vi "SaveStatMeas.vi"(2 "Min":dbl, 3 "Max":dbl, 4 "error in":errorcluster, 5 "Ecart Type":dbl, 6 "Moyenne":dbl, 7 "storage refnum (file)":refnum<k20>) -> (0 "error out":errorcluster, 1 "storage refnum (file) 2":refnum<k20>)   [LabVIEW 2014]
uses:
  <vilib>/Platform/storage/Storage.llb/usiSequenceRepresentation.ctl
  <vilib>/Platform/storage/Storage.llb/usiOverwriteOptions.ctl
  <vilib>/Platform/storage/lvStorage.llb/_createOrGetByNameExplicitChildObject.vi
  <vilib>/Platform/storage/Storage.llb/__savePropString.vi
  <vilib>/Platform/storage/lvStorage.llb/xStorage/xStorageSupp/ErrorOut.vi
  <vilib>/Platform/storage/lvStorage.llb/__saveFloat64Channel.vi
  <vilib>/Platform/storage/lvStorage.llb/xStorage/Write Data/Write Data.xnode
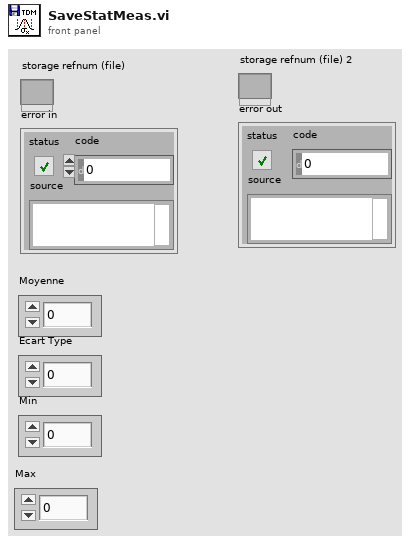
[diagram p1: front panel]
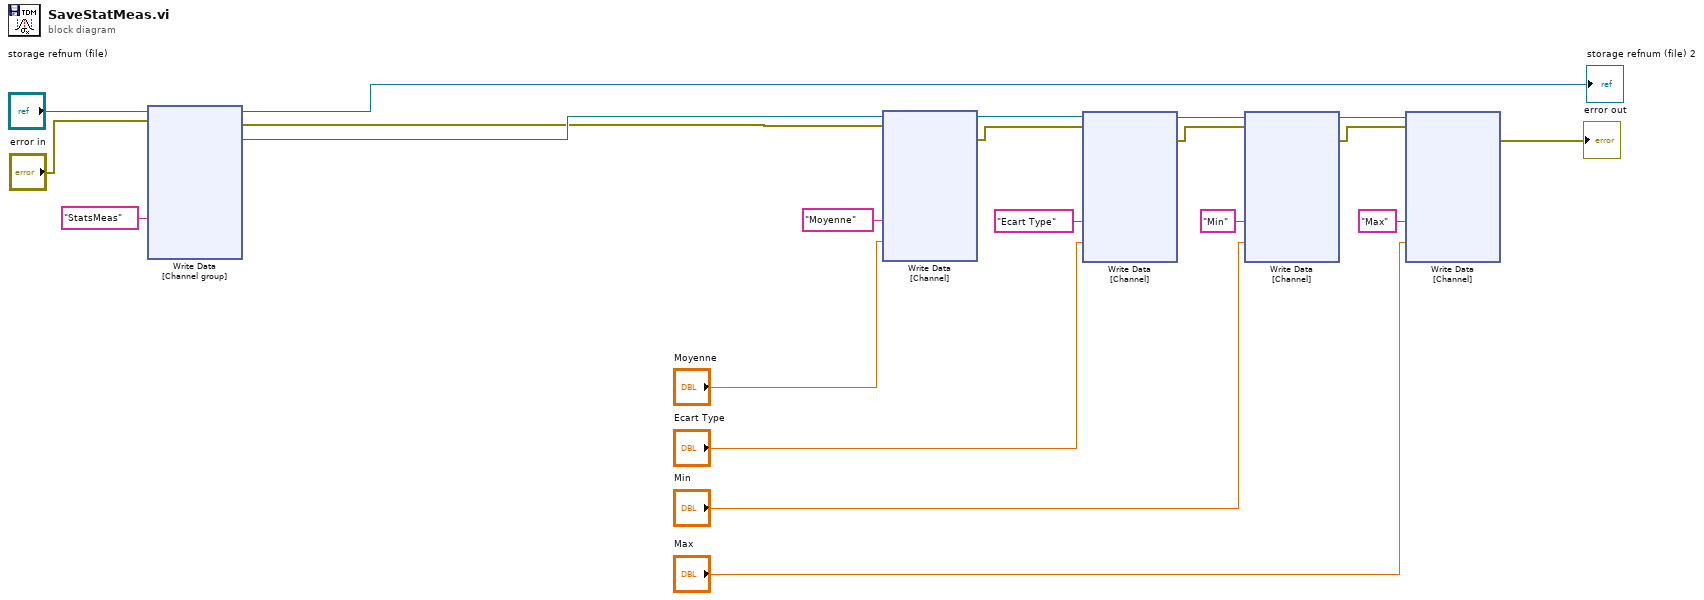
[diagram p0: block diagram]
diagram:
  n1 = xnode "Write Data\n[Channel group]"("Name"="StatsMeas", "storage refnum (file)"="storage refnum (file)", "error in"="error in") -> ("error out"=w17:errorcluster, "storage refnum (channel group)"=w18:refnum<k20>)  [unwired: 1 in, 1 out]
  n2 = xnode "Write Data\n[Channel]"("Name"="Moyenne", "Signal"="Moyenne", "storage refnum (channel group)"=w18, "error in"=w17) -> ("storage refnum (channel group) out"=w11:refnum<k20>, "error out"=w14:errorcluster)  [unwired: 2 in, 1 out]
  n3 = xnode "Write Data\n[Channel]"("Name"="Ecart Type", "Signal"="Ecart Type", "storage refnum (channel group)"=w11, "error in"=w14) -> ("storage refnum (channel group) out"=w10:refnum<k20>, "error out"=w9:errorcluster)  [unwired: 2 in, 1 out]
  n4 = xnode "Write Data\n[Channel]"("Name"="Min", "Signal"="Min", "storage refnum (channel group)"=w10, "error in"=w9) -> ("storage refnum (channel group) out"=w4:refnum<k20>, "error out"=w3:errorcluster)  [unwired: 2 in, 1 out]
  n5 = xnode "Write Data\n[Channel]"("Name"="Max", "Signal"="Max", "storage refnum (channel group)"=w4, "error in"=w3) -> ("error out"=→"error out":errorcluster)  [unwired: 2 in, 2 out]
  "storage refnum (file) 2" <- "storage refnum (file)"
